vi "GetButton.vi"(10 "sensors list":string[](array[string]), 11 "packet in":u8[](array[numeric])) -> (3 "button state":bool)   [LabVIEW 2018]
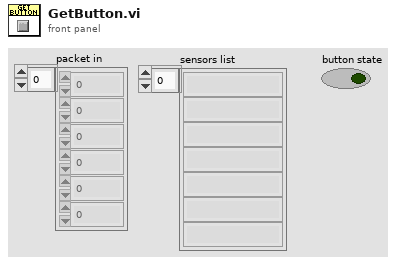
[diagram p1: front panel]
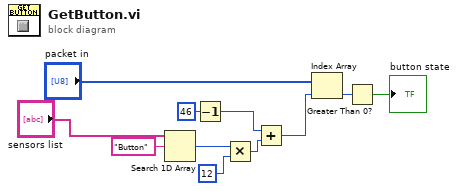
[diagram p0: block diagram]
diagram:
  n1 = Search 1D Array(1D array="sensors list", element="Button") -> (index of element=w5:i32)  [unwired: 1 in]
  n2 = Decrement(x=46) -> (x-1=w7:i32)
  n3 = Multiply(x=w5, y=12) -> (x*y=w6:i32)
  n4 = Add(x=w7, y=w6) -> (x+y=w9:i32)
  n5 = Index Array(array="packet in", index=w9) -> (element=w10:u8)
  n6 = Greater Than 0?(x=w10) -> (x > 0?=→"button state":bool)
